vi "Command_Drive_Straight.vi"(7 "Startup":bool, 8 "Parameter 4":dbl, 9 "Parameter 3":dbl, 10 "Parameter 2":dbl, 11 "Parameter 1":dbl) -> (2 "Left":dbl, 3 "Right":dbl, 4 "Reint":bool, 6 "Completed":bool)   [LabVIEW 2019]
uses:
  Auto Utilities/Command_Execution_State.ctl
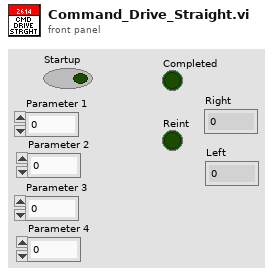
[diagram p1: front panel]
types:
  T1 = typedef "Command_Execution_State.ctl" = enum16{"Initialize", "Execute", "Finish"}
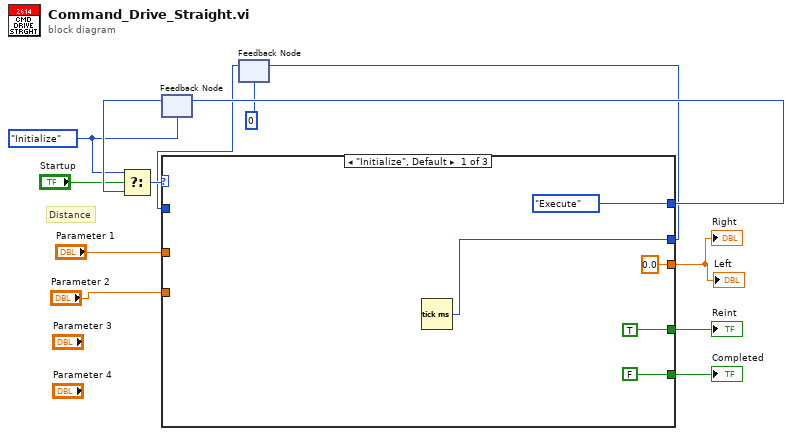
[diagram p0: block diagram]
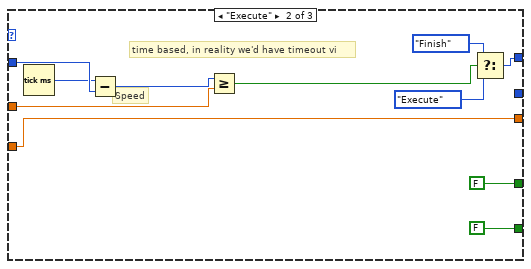
[diagram p2: hidden frame]
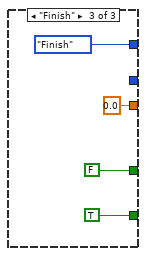
[diagram p3: hidden frame]
diagram:
  w7 = Command_Execution_State."Initialize" ("Play State")
  # "Distance"
  n1 = feedback #1(w7) -> (w11:T1)
  n2 = Select(t=w7, s="Startup", f=w11) -> (s? t:f=w13:T1)
  n3 = feedback #2(u32 0 ("millisecond timer value")) -> (w3:u32)
  n4 = case shown="\"Initialize\", Default" w13 {
    tunnel: [Command_Execution_State."Execute" ("Play State") w23 Command_Execution_State."Finish" ("Play State")] -> w12
    tunnel: [FALSE FALSE TRUE] -> w10
    tunnel: [TRUE FALSE FALSE] -> w8
    tunnel: "Parameter 2" -> [_ w27 _]
    tunnel: [0.0 ("Parameter 2") w27 0.0 ("Parameter 2")] -> w5
    tunnel: [w14 _ _] -> w4
    tunnel: w3 -> [_ w26 _]
    tunnel: "Parameter 1" -> [_ w24 _]
    frame "Initialize", Default {
      n5 = Tick Count (ms)() -> (millisecond timer value=w14:u32)
    }
    frame "Execute" {
      # "Speed"
      # "time based, in reality we'd have timeout vi"
      n6 = Tick Count (ms)() -> (millisecond timer value=w19:u32)
      n7 = Subtract(x=w19, y=w26) -> (x-y=w25:u32)
      n8 = Greater Or Equal?(x=w25, y=w24) -> (x >= y?=w21:bool)
      n9 = Select(t=Command_Execution_State."Finish" ("Play State"), s=w21, f=Command_Execution_State."Execute" ("Play State")) -> (s? t:f=w23:T1)
    }
    frame "Finish" {
    }
  }
  "Completed" <- w10
  "Reint" <- w8
  "Left" <- w5
  "Right" <- w5
  n10 = feedback-in #1(w12) -> ()
  n11 = feedback-in #2(w4) -> ()
